vi "CheckSumm (SubVI).vi"(11 "Input String":string=":01E2000000000000000F") -> (1 "CheckSumm":string, 2 "CheckSumm_U32":u32, 3 "length":i32, 4 "Array":u8[](array[numeric]) format="%x")   [LabVIEW 2017, in "LV_Unicorn.lvlib"]
uses:
  LV_Unicorn.lvlib
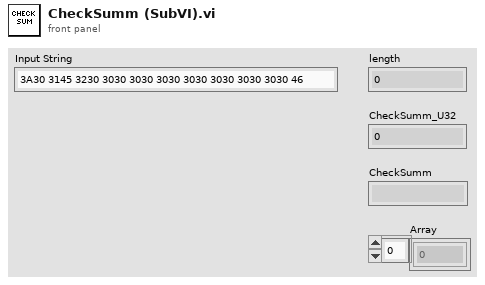
[diagram p1: front panel]
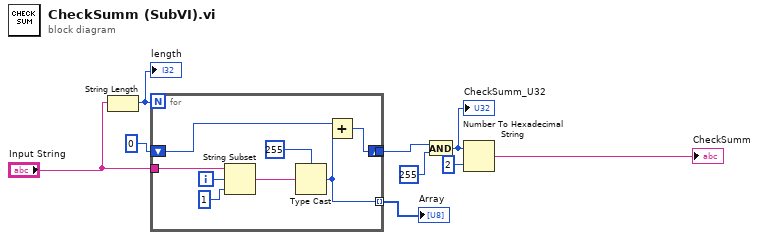
[diagram p0: block diagram]
diagram:
  n1 = String Length(string="Input String") -> (length=w2:i32)
  "length" <- w2
  n2 = for {
    N: w2 -> [_]
    tunnel: "Input String" -> [w15]
    tunnel: [w12] -> w4 mode=indexing
    shift-right: [w10] -> w9
    shift-left: u8 0 -> [w11]
    tunnel: [w10] -> _
    i -> [w16]
    n3 = String Subset(string=w15, offset (0)=w16, length (rest)=1 ("length (rest)")) -> (substring=w13:string)
    n4 = Type Cast(type=u8 255, x=w13) -> (*(type *) &x=w12:u8)
    n5 = Add(x=w11, y=w12) -> (x+y=w10:u8)
  }
  "Array" <- w4
  n6 = And(x=w9, y=u32 255) -> (x .and. y?=w7:u32)
  "CheckSumm_U32" <- w7
  n7 = Number To Hexadecimal String(1:i16 2 ("width (-)"), 2:w7) -> (0:→"CheckSumm":string)
